vi "getPaths.vi"(8 "Error In":errorcluster) -> (0 "Error Out":errorcluster, 3 "Application Path Cluster":T1)   [LabVIEW 2018]
uses:
  controls/pathCluster.ctl
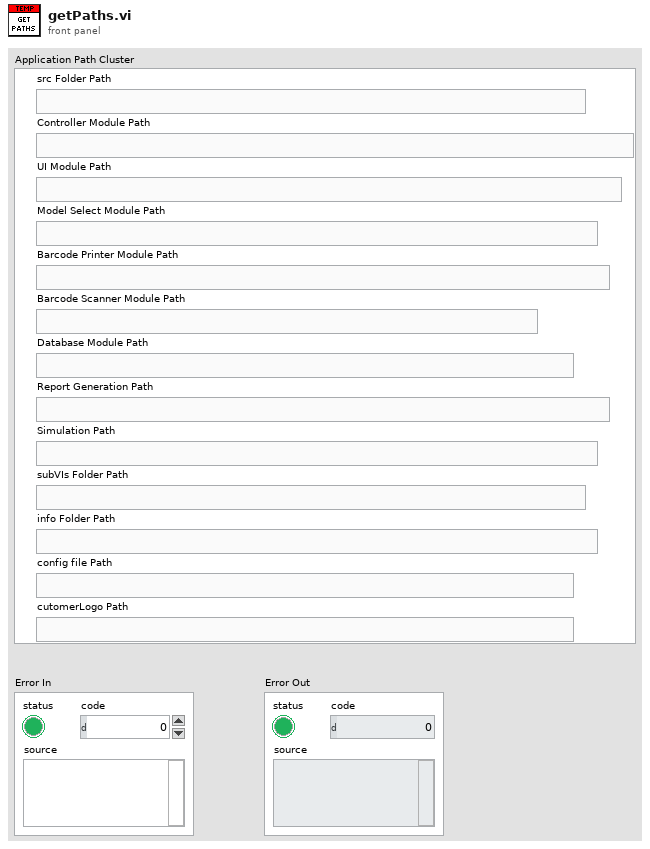
[diagram p1: front panel]
types:
  T1 = typedef "pathCluster.ctl" = cluster{"src Folder Path":path, "Controller Module Path":path, "UI Module Path":path, "Model Select Module Path":path, "Barcode Printer Module Path":path, "Barcode Scanner Module Path":path, "Database Module Path":path, "Report Generation Path":path, "Simulation Path":path, "subVIs Folder Path":path, "info Folder Path":path, "config file Path":path, "cutomerLogo Path":path}
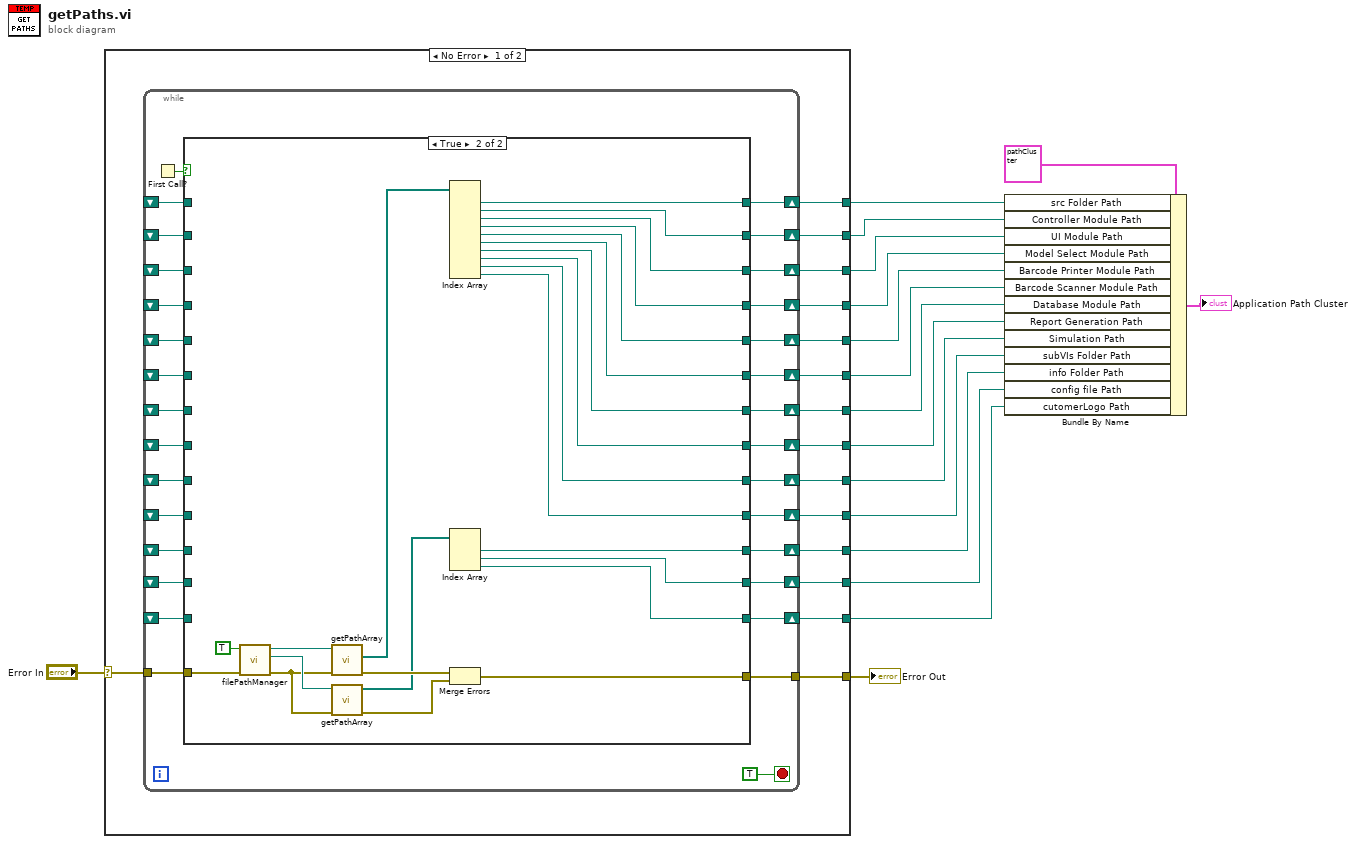
[diagram p0: block diagram]
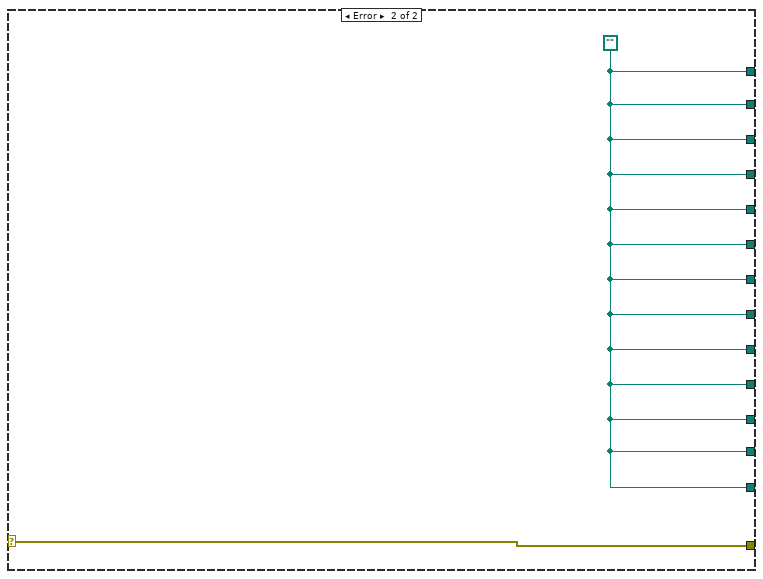
[diagram p3: hidden frame]
diagram:
  n1 = case shown="No Error" "Error In" {
    selector: "Error In" -> [w32 w101]
    tunnel: [w31 w101] -> w1
    tunnel: [w30 w100] -> w16
    tunnel: [w29 w100] -> w15
    tunnel: [w28 w100] -> w13
    tunnel: [w27 w100] -> w12
    tunnel: [w26 w100] -> w10
    tunnel: [w25 w100] -> w9
    tunnel: [w24 w100] -> w8
    tunnel: [w23 w100] -> w7
    tunnel: [w22 w100] -> w6
    tunnel: [w21 w100] -> w5
    tunnel: [w20 w100] -> w4
    tunnel: [w19 w100] -> w3
    tunnel: [w18 w100] -> w11
    frame No Error {
      n2 = while {
        tunnel: w32 -> [w62]
        tunnel: [w61] -> w31
        shift-right: [w59] -> w30
        shift-left: _ -> [w57]
        shift-right: [w58] -> w29
        shift-left: _ -> [w56]
        shift-right: [w55] -> w28
        shift-left: _ -> [w54]
        shift-right: [w53] -> w27
        shift-left: _ -> [w52]
        shift-right: [w50] -> w26
        shift-left: _ -> [w42]
        shift-right: [w49] -> w25
        shift-left: _ -> [w41]
        shift-right: [w48] -> w24
        shift-left: _ -> [w40]
        shift-right: [w47] -> w23
        shift-left: _ -> [w39]
        shift-right: [w46] -> w22
        shift-left: _ -> [w38]
        shift-right: [w45] -> w21
        shift-left: _ -> [w37]
        shift-right: [w51] -> w20
        shift-left: _ -> [w36]
        shift-right: [w44] -> w19
        shift-left: _ -> [w35]
        shift-right: [w43] -> w18
        shift-left: _ -> [w34]
        stop <- TRUE stop-if-true
        n3 = First Call?() -> (First Call?: T/F=w60:bool)
        n4 = case shown="True" w60 {
          tunnel: w62 -> [w76 w99]
          tunnel: [w76 w93] -> w61
          tunnel: [w75 w89] -> w59
          tunnel: [w74 w88] -> w58
          tunnel: w57 -> [w75 _]
          tunnel: w56 -> [w74 _]
          tunnel: [w73 w87] -> w55
          tunnel: w54 -> [w73 _]
          tunnel: [w72 w86] -> w53
          tunnel: w52 -> [w72 _]
          tunnel: [w65 w79] -> w51
          tunnel: [w71 w85] -> w50
          tunnel: [w70 w84] -> w49
          tunnel: [w69 w83] -> w48
          tunnel: [w68 w82] -> w47
          tunnel: [w67 w81] -> w46
          tunnel: [w66 w80] -> w45
          tunnel: [w64 w78] -> w44
          tunnel: [w63 w77] -> w43
          tunnel: w42 -> [w71 _]
          tunnel: w41 -> [w70 _]
          tunnel: w40 -> [w69 _]
          tunnel: w39 -> [w68 _]
          tunnel: w38 -> [w67 _]
          tunnel: w37 -> [w66 _]
          tunnel: w36 -> [w65 _]
          tunnel: w35 -> [w64 _]
          tunnel: w34 -> [w63 _]
          frame False {
          }
          frame True {
            n5 = call "filePathManager.vi"("Error In"=w99, "First Call?"=TRUE) -> ("Error Out"=w94:errorcluster, "info File Path"=w95:path, "src File Path"=w97:path)  [unwired: 7 in]
            n6 = call "getPathArray.vi"("Error In"=w94, "File Path"=w97) -> ("Error Out"=w96:errorcluster, "Folder Path Array"=w91:path[])  [unwired: 7 in, 1 out]
            n7 = call "getPathArray.vi"("Error In"=w94, "File Path"=w95) -> ("Error Out"=w92:errorcluster, "File Path Array"=w90:path[])  [unwired: 7 in, 1 out]
            n8 = Index Array(array=w91) -> (element #1=w89:path, element #2=w88:path, element #3=w87:path, element #4=w86:path, element #5=w85:path, element #6=w84:path, element #7=w83:path, element #8=w82:path, element #9=w81:path, element #10=w80:path)  [unwired: 10 in]
            n9 = Index Array(array=w90) -> (element #1=w79:path, element #2=w78:path, element #3=w77:path)  [unwired: 3 in]
            n10 = Merge Errors(w96, w92) -> (w93:errorcluster)
          }
        }
      }
    }
    frame Error {
      w100 = path ""
    }
  }
  "Error Out" <- w1
  n11 = Bundle By Name(cluster=T1 {"src Folder Path"=path "", "Controller Module Path"=path "", "UI Module Path"=path "", "Model Select Module Path"=path "", "Barcode Printer Module Path"=path "", "Barcode Scanner Module Path"=path "", "Database Module Path"=path "", "Report Generation Path"=path "", "Simulation Path"=path "", "subVIs Folder Path"=path "", "info Folder Path"=path "", "config file Path"=path "", "cutomerLogo Path"=path ""} ("Path Cluster"), "src Folder Path"=w16, "Controller Module Path"=w15, "UI Module Path"=w13, "Model Select Module Path"=w12, "Barcode Printer Module Path"=w10, "Barcode Scanner Module Path"=w9, "Database Module Path"=w8, "Report Generation Path"=w7, "Simulation Path"=w6, "subVIs Folder Path"=w5, "info Folder Path"=w4, "config file Path"=w3, "cutomerLogo Path"=w11) -> (→"Application Path Cluster":T1)
